vi "CompatabilityTesting.vi"() -> ()   [LabVIEW 2019]
uses:
  subVIs/typedefs/Parsed Path - Cluster.ctl
  <vilib>/Analysis/Matrix/Datatypes/RealMatrix.ctl
  subVIs/typedefs/Parsed Funnel - Cluster.ctl
  subVIs/typedefs/Parsed Rect - Cluster.ctl
  Dot/Dot.lvclass
  ParseVectorFile/ParseVectorFile.lvclass
  C:/Program Files (x86)/National Instruments/LabVIEW 2019/vi.lib/JKI/JKI SMO/SMO/SMO.lvclass
  <vilib>/JKI/JKI SMO/SMO/SMO.lvclass
  <vilib>/Analysis/Matrix/NI_Matrix.lvlib
panel:
  out "Parsing Data 2":T5
  out "Image Size":cluster{"Width":dbl, "Height":dbl}
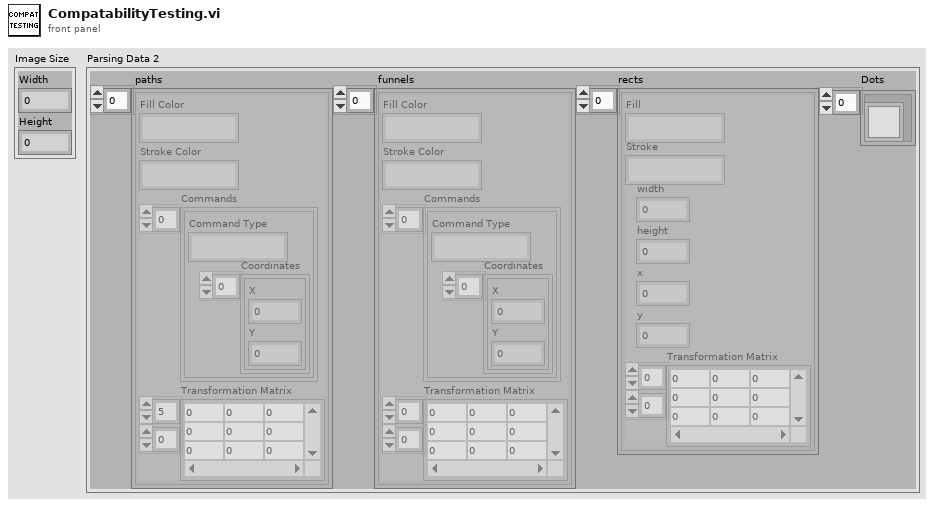
[diagram p1: front panel]
types:
  T1 = typedef "Parsed Path - Cluster.ctl" = cluster{"Fill Color":string, "Stroke Color":string, "Commands":cluster{"Command Type":string, "Coordinates":cluster{"X":dbl, "Y":dbl}[]}[], "Transformation Matrix":T2}
  T2 = typedef "NI_Matrix.lvlib/RealMatrix.ctl" = dbl[][]
  T3 = typedef "Parsed Funnel - Cluster.ctl" = cluster{"Fill Color":string, "Stroke Color":string, "Commands":cluster{"Command Type":string, "Coordinates":cluster{"X":dbl, "Y":dbl}[]}[], "Transformation Matrix":T2}
  T4 = typedef "Parsed Rect - Cluster.ctl" = cluster{"Fill":string, "Stroke":string, "width":dbl, "height":dbl, "x":dbl, "y":dbl, "Transformation Matrix":T2}
  T5 = cluster{" paths":T1[], " funnels":T3[], "rects":T4[], "Dots":refnum<class "Dot.lvclass">[]}
  T6 = typedef "ParseVectorFile.lvclass/PublicEvents--ParseVectorFile.ParsedData.ctl" = cluster{"Paths":refnum<class "Path.lvclass">[], "Rectangles":refnum<class "Rectangle.lvclass">[], "SVGImage":refnum<class "SVGImage.lvclass">, "Dots":refnum<class "Dot.lvclass">[]}
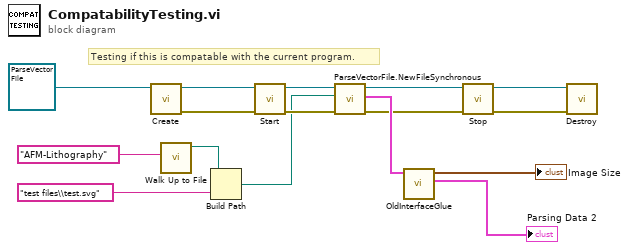
[diagram p0: block diagram]
diagram:
  # "Testing if this is compatable with the current program."
  n1 = call <vilib>:"Create.vi"("SMO"=refnum<class "ParseVectorFile.lvclass"> refnum ("ParseVectorFile.lvclass")) -> ("error out"=w9:errorcluster, "SMO out"=w10:refnum<class "ParseVectorFile.lvclass">)  [unwired: 8 in, 1 out]
  n2 = call "Walk Up to File.vi"("name or relative path"="AFM-Lithography" ("NewFile")) -> ("File Path"=w12:path)  [unwired: 8 in, 2 out]
  n3 = Build Path(base path=w12, name or relative path="test files\\test.svg" ("NewFile")) -> (appended path=w1:path)
  n4 = call <vilib>:"Start.vi"("error in (no error)"=w9, "SMO"=w10) -> ("error out"=w4:errorcluster, "SMO out"=w6:refnum<class "ParseVectorFile.lvclass">)  [unwired: 8 in]
  n5 = call "ParseVectorFile.NewFileSynchronous.vi"("error in (no error)"=w4, "Path"=w1, "ParseVectorFile"=w6) -> ("error out"=w3:errorcluster, "ParsedData"=w16:T6, "ParseVectorFile out"=w5:refnum<class "ParseVectorFile.lvclass">)  [unwired: 6 in]
  n6 = call "OldInterfaceGlue.vi"("ParsedData"=w16) -> ("Parsing Data"=→"Parsing Data 2":T5, "Image Size"=→"Image Size":cluster{"Width":dbl, "Height":dbl})  [unwired: 8 in, 1 out]
  n7 = call <vilib>:"Stop.vi"("error in (no error)"=w3, "SMO"=w5) -> ("error out"=w7:errorcluster, "SMO out"=w8:refnum<class "ParseVectorFile.lvclass">)  [unwired: 8 in]
  n8 = call <vilib>:"Destroy.vi"("error in (no error)"=w7, "SMO"=w8) -> ()  [unwired: 9 in, 1 out]
